vi "mxwScript_API_Option_UseLibrariesToSave.vi"(0 "options in":T2[](array[typedef]), 1 "IconPath":path, 2 "SaveInLibrary":T1=enum."Never", 5 "Name":string, 7 "DisplayName":string, 9 "Description":string, 11 "error in (no error)":errorcluster, 12 "HelpPath":path, 13 "HelpTag":string) -> (4 "options out":T2[](array[typedef]), 15 "error out":errorcluster)   [LabVIEW 2017]
doc: "Sets the default relationship between the template and block diagram reference points. This is used to calculate the drop position of templates."
uses:
  codeGenAPISupport.llb/cgAPI_mxwScript_OptionData.ctl
  codeGenAPISupport.llb/cgAPI_mxwScript_Save_SaveInLibraryOptions.ctl
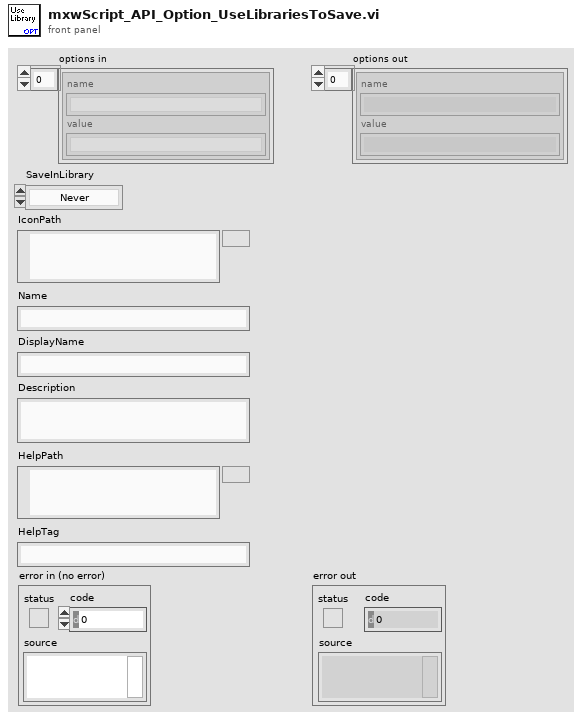
[diagram p1: front panel]
types:
  T1 = typedef "cgAPI_mxwScript_Save_SaveInLibraryOptions.ctl" = enum16{"Always", "Never", "IfSubVIs"}
  T2 = typedef "cgAPI_mxwScript_OptionData.ctl" = cluster{"name":string, "value":string}
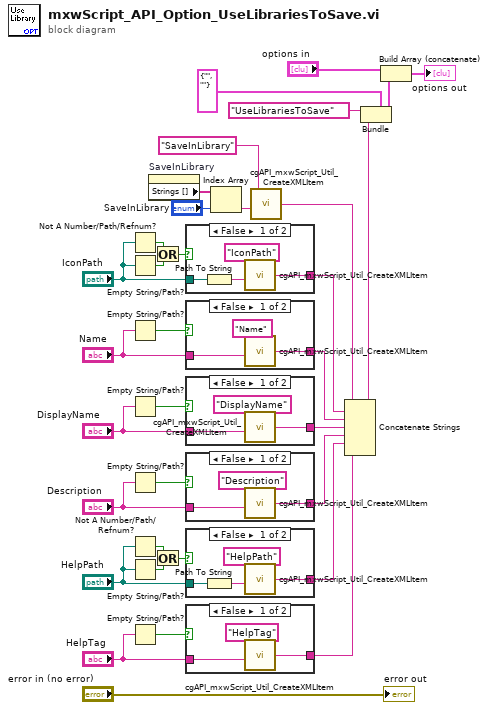
[diagram p0: block diagram]
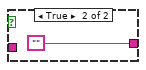
[diagram p2: hidden frame]
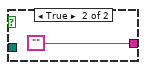
[diagram p3: hidden frame]
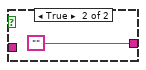
[diagram p4: hidden frame]
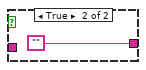
[diagram p5: hidden frame]
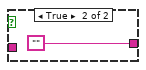
[diagram p6: hidden frame]
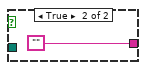
[diagram p7: hidden frame]
diagram:
  n1 = Not A Number/Path/Refnum?(number/path/refnum="IconPath") -> (NaN/Path/Refnum?=w20:bool)
  n2 = Empty String/Path?(string/path="IconPath") -> (empty?=w19:bool)
  n3 = Empty String/Path?(string/path="Name") -> (empty?=w17:bool)
  n4 = Empty String/Path?(string/path="DisplayName") -> (empty?=w15:bool)
  n5 = Empty String/Path?(string/path="Description") -> (empty?=w13:bool)
  n6 = Not A Number/Path/Refnum?(number/path/refnum="HelpPath") -> (NaN/Path/Refnum?=w10:bool)
  n7 = Empty String/Path?(string/path="HelpPath") -> (empty?=w11:bool)
  n8 = Empty String/Path?(string/path="HelpTag") -> (empty?=w7:bool)
  n9 = property on="SaveInLibrary" class="Enum (strict)"() -> ("Strings []"=w28:string[])  [unwired: 2 in, 2 out]
  n10 = Or(x=w20, y=w19) -> (x .or. y?=w21:bool)
  n11 = Or(x=w10, y=w11) -> (x .or. y?=w9:bool)
  n12 = case shown="False" w21 {
    tunnel: "IconPath" -> [w38 _]
    tunnel: [w35 ""] -> w22
    frame False {
      n13 = Path To String(path=w38) -> (string=w37:string)
      n14 = call "cgAPI_mxwScript_Util_CreateXMLItem.vi"("value"=w37, "tag"="IconPath") -> ("item"=w35:string)  [unwired: 4 out]
    }
    frame True {
    }
  }
  n15 = case shown="False" w17 {
    tunnel: "Name" -> [w40 _]
    tunnel: [w41 ""] -> w16
    frame False {
      n16 = call "cgAPI_mxwScript_Util_CreateXMLItem.vi"("value"=w40, "tag"="Name") -> ("item"=w41:string)  [unwired: 4 out]
    }
    frame True {
    }
  }
  n17 = case shown="False" w15 {
    tunnel: "DisplayName" -> [w44 _]
    tunnel: [w45 ""] -> w5
    frame False {
      n18 = call "cgAPI_mxwScript_Util_CreateXMLItem.vi"("value"=w44, "tag"="DisplayName") -> ("item"=w45:string)  [unwired: 4 out]
    }
    frame True {
    }
  }
  n19 = case shown="False" w13 {
    tunnel: "Description" -> [w48 _]
    tunnel: [w49 ""] -> w3
    frame False {
      n20 = call "cgAPI_mxwScript_Util_CreateXMLItem.vi"("value"=w48, "tag"="Description") -> ("item"=w49:string)  [unwired: 4 out]
    }
    frame True {
    }
  }
  n21 = case shown="False" w9 {
    tunnel: "HelpPath" -> [w55 _]
    tunnel: [w52 ""] -> w2
    frame False {
      n22 = Path To String(path=w55) -> (string=w54:string)
      n23 = call "cgAPI_mxwScript_Util_CreateXMLItem.vi"("value"=w54, "tag"="HelpPath") -> ("item"=w52:string)  [unwired: 4 out]
    }
    frame True {
    }
  }
  n24 = case shown="False" w7 {
    tunnel: "HelpTag" -> [w57 _]
    tunnel: [w58 ""] -> w4
    frame False {
      n25 = call "cgAPI_mxwScript_Util_CreateXMLItem.vi"("value"=w57, "tag"="HelpTag") -> ("item"=w58:string)  [unwired: 4 out]
    }
    frame True {
    }
  }
  n26 = Index Array(array=w28, index="SaveInLibrary") -> (element=w26:string)
  n27 = call "cgAPI_mxwScript_Util_CreateXMLItem.vi"("value"=w26, "tag"="SaveInLibrary") -> ("item"=w24:string)  [unwired: 4 out]
  n28 = Concatenate Strings(w24, w22, w16, w5, w3, w2, w4) -> (w1:string)
  n29 = Bundle(cluster=T2 {"name"="", "value"=""} ("optionData"), "name"="UseLibrariesToSave", "value"=w1) -> (w32:T2)
  n30 = Build Array (concatenate)("options in", w32) -> (→"options out":T2[])
  "error out" <- "error in (no error)"
